vi "ep_Check Analog Channel Validation.vi"(8 "error in (no error)":errorcluster, 11 "analog channel info in":T1[](array[typedef])) -> (0 "error out":errorcluster, 3 "analog channel info out":T1[](array[typedef]))   [LabVIEW 2011, in "NI_EP_COMTRADE.lvlib"]
uses:
  <vilib>/addons/Electrical Power/File IO/NI_EP_COMTRADE.lvlib
  <vilib>/addons/Electrical Power/File IO/COMTRADE/typedefs/ep_Analog Channel Info (UI).ctl
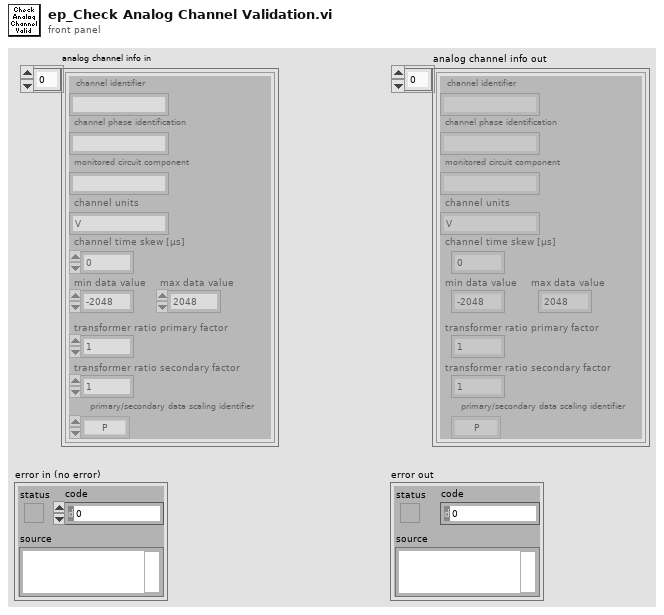
[diagram p1: front panel]
types:
  T1 = typedef "NI_EP_COMTRADE.lvlib/ep_Analog Channel Info (UI).ctl" = cluster{"channel identifier":string, "channel phase identification":string, "monitored circuit component":string, "channel units":string, "channel time skew [µs]":sgl, "min data value":sgl, "max data value":sgl, "transformer ratio primary factor":sgl, "transformer ratio secondary factor":sgl, "primary/secondary data scaling identifier":enum16{"P", "S"}}
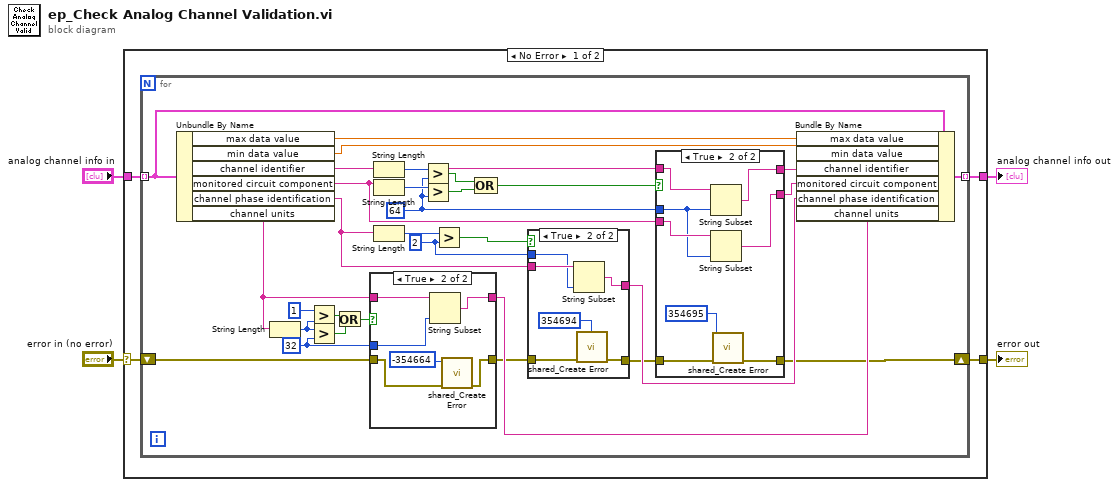
[diagram p0: block diagram]
diagram:
  n1 = case shown="No Error" "error in (no error)" {
    selector: "error in (no error)" -> [w7 w68]
    tunnel: [w6 w68] -> w3
    tunnel: "analog channel info in" -> [w8 w67]
    tunnel: [w5 w67] -> w1
    frame No Error {
      n2 = for {
        tunnel: w8 -> [w25] mode=indexing
        shift-right: [w9] -> w6
        shift-left: w7 -> [w26]
        tunnel: [w22] -> w5 mode=indexing
        w30 = 32 ("y")
        w10 = 2 ("y")
        w32 = 64 ("y")
        n3 = Unbundle By Name(w25) -> ("max data value"=w21:sgl, "min data value"=w20:sgl, "channel identifier"=w34:string, "monitored circuit component"=w33:string, "channel phase identification"=w15:string, "channel units"=w27:string)
        n4 = String Length(string=w27) -> (length=w29:i32)
        n5 = Greater?(x=1, y=w29) -> (0:w19:bool)
        n6 = Greater?(x=w29, y=w30) -> (0:w18:bool)
        n7 = Or(x=w19, y=w18) -> (x .or. y?=w17:bool)
        n8 = case shown="True" w17 {
          tunnel: w30 -> [_ w55]
          tunnel: w27 -> [w49 w54]
          tunnel: [w49 w53] -> w16
          tunnel: w26 -> [w48 w52]
          tunnel: [w48 w50] -> w13
          frame False {
          }
          frame True {
            n9 = String Subset(string=w54, length (rest)=w55) -> (substring=w53:string)  [unwired: 1 in]
            n10 = call <vilib>:"shared_Create Error.vi"("error in (no error)"=w52, "error code (0)"=-354664 ("code")) -> ("error out"=w50:errorcluster)  [unwired: 9 in]
          }
        }
        n11 = String Length(string=w34) -> (length=w39:i32)
        n12 = String Length(string=w33) -> (length=w38:i32)
        n13 = String Length(string=w15) -> (length=w31:i32)
        n14 = Greater?(x=w39, y=w32) -> (0:w37:bool)
        n15 = Greater?(x=w38, y=w32) -> (0:w36:bool)
        n16 = Greater?(x=w31, y=w10) -> (0:w11:bool)
        n17 = Compound Arithmetic op=OR(w37, w36) -> (w35:bool)
        n18 = case shown="True" w11 {
          tunnel: [w41 w47] -> w12
          tunnel: w13 -> [w41 w45]
          tunnel: w10 -> [_ w42]
          tunnel: w15 -> [w40 w44]
          tunnel: [w40 w43] -> w14
          frame False {
          }
          frame True {
            n19 = String Subset(string=w44, length (rest)=w42) -> (substring=w43:string)  [unwired: 1 in]
            n20 = call <vilib>:"shared_Create Error.vi"("error in (no error)"=w45, "error code (0)"=354694 ("code")) -> ("error out"=w47:errorcluster)  [unwired: 9 in]
          }
        }
        n21 = case shown="True" w35 {
          tunnel: w34 -> [w58 w66]
          tunnel: w33 -> [w57 w65]
          tunnel: w32 -> [_ w64]
          tunnel: w12 -> [w56 w61]
          tunnel: [w58 w63] -> w24
          tunnel: [w57 w62] -> w23
          tunnel: [w56 w60] -> w9
          frame False {
          }
          frame True {
            n22 = String Subset(string=w66, length (rest)=w64) -> (substring=w63:string)  [unwired: 1 in]
            n23 = String Subset(string=w65, length (rest)=w64) -> (substring=w62:string)  [unwired: 1 in]
            n24 = call <vilib>:"shared_Create Error.vi"("error in (no error)"=w61, "error code (0)"=354695 ("code")) -> ("error out"=w60:errorcluster)  [unwired: 9 in]
          }
        }
        n25 = Bundle By Name(cluster=w25, "max data value"=w21, "min data value"=w20, "channel identifier"=w24, "monitored circuit component"=w23, "channel phase identification"=w14, "channel units"=w16) -> (w22:T1)
      }
    }
    frame Error {
    }
  }
  "error out" <- w3
  "analog channel info out" <- w1
